vi "test.vi"() -> ()   [LabVIEW 2018]
panel:
  out "read buffer":string
  in  "VISA resource name":refnum<visa-resource-name>
  out "error out":errorcluster
  in  "error in (no error)":errorcluster
  in  "Write buffer":string
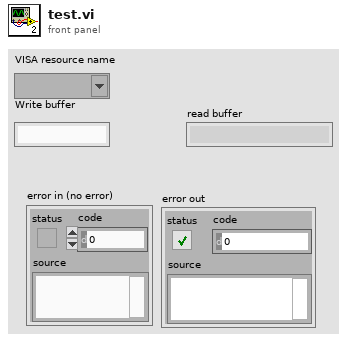
[diagram p1: front panel]
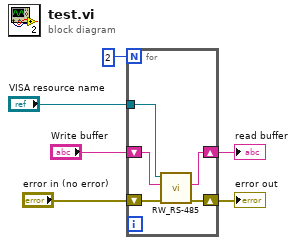
[diagram p0: block diagram]
diagram:
  n1 = for {
    N: 2 -> [_]
    tunnel: "VISA resource name" -> [w11]
    shift-right: [w8] -> w3
    shift-left: "Write buffer" -> [w10]
    shift-right: [w7] -> w2
    shift-left: "error in (no error)" -> [w9]
    n2 = call "RW_RS-485.vi"("error in (no error)"=w9, "Initial Command"=w10, "VISA Refnum in"=w11) -> ("error out"=w7:errorcluster, "read buffer"=w8:string)  [unwired: 7 in]
  }
  "read buffer" <- w3
  "error out" <- w2
